vi "Read Spot Measurement.vi"(8 "error in (no error)":errorcluster, 9 "Measurement Type (0: Charge)":i32(ring) items=["Charge", "Current", "Resistance", "Voltage"], 10 "Channel (1: Channel 1)":i32(ring)=1 items=["Channel 1"=1], 11 "VISA resource name":refnum<visa-resource-name>) -> (0 "error out":errorcluster, 2 "Measurement":dbl, 3 "VISA resource name out":refnum<visa-resource-name>)   [LabVIEW 2012, in "Keysight B2980 Series.lvlib"]
doc: "Executes a spot (one-shot) measurement and returns the measurement result data."
uses:
  Keysight B2980 Series.lvlib
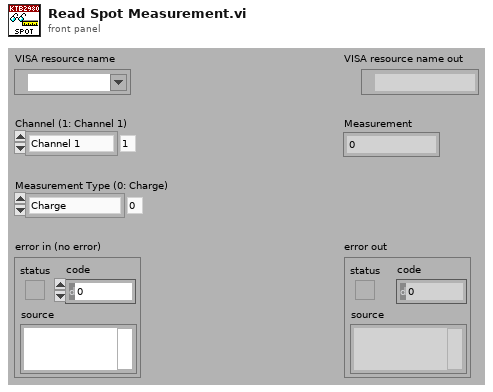
[diagram p1: front panel]
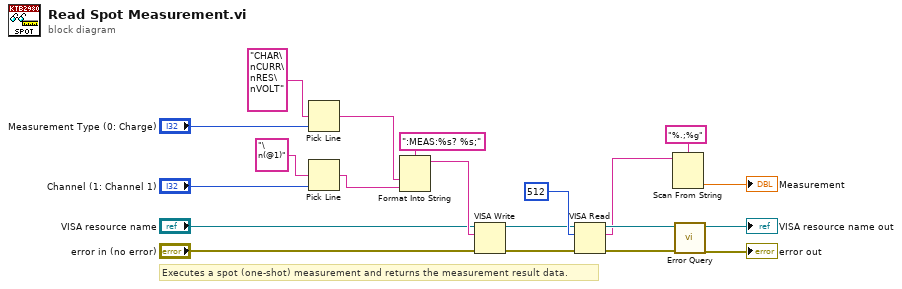
[diagram p0: block diagram]
diagram:
  # "Executes a spot (one-shot) measurement and returns the measurement result data."
  n1 = Pick Line(multi-line string="CHAR\nCURR\nRES\nVOLT", line index="Measurement Type (0: Charge)") -> (output string=w17:string)  [unwired: 1 out]
  n2 = Pick Line(multi-line string="\n(@1)", line index="Channel (1: Channel 1)") -> (output string=w4:string)  [unwired: 1 out]
  n3 = Format Into String(format string=":MEAS:%s? %s;", w17, w4) -> (resulting string=w16:string)  [unwired: 2 in, 1 out]
  n4 = VISA Write(VISA resource name="VISA resource name", write buffer=w16, error in (no error)="error in (no error)") -> (VISA resource name out=w12:refnum<visa-resource-name>, error out=w11:errorcluster)  [unwired: 1 out]
  n5 = VISA Read(VISA resource name=w12, byte count=u32 512, error in (no error)=w11) -> (VISA resource name out=w10:refnum<visa-resource-name>, read buffer=w3:string, error out=w9:errorcluster)  [unwired: 1 out]
  n6 = Scan From String(format string="%.;%g", input string=w3) -> (output 1=→"Measurement":dbl)  [unwired: 2 in, 4 out]
  n7 = call "Error Query.vi"("error in (no error)"=w9, "VISA resource name"=w10) -> ("error out"=→"error out":errorcluster, "VISA resource name out"=→"VISA resource name out":refnum<visa-resource-name>)  [unwired: 8 out]
